vi "P1.vi"() -> ()   [LabVIEW 2019]
panel:
  out "A-B":dbl
  out "A+B":dbl
  in  "B":dbl
  in  "A":dbl
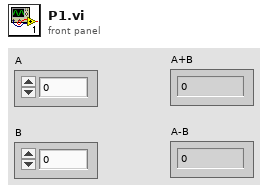
[diagram p1: front panel]
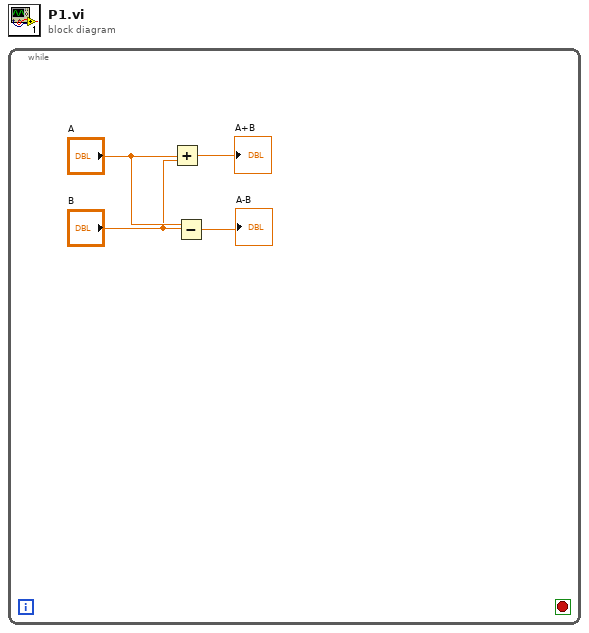
[diagram p0: block diagram]
diagram:
  n1 = while {
    stop <- _ stop-if-true
    n2 = Add(x="A", y="B") -> (x+y=→"A+B":dbl)
    n3 = Subtract(x="A", y="B") -> (x-y=→"A-B":dbl)
  }
